vi "QMH-Check Loop Error.vi"(6 "Exit on Error? (F)":bool, 9 "Ignore Errors":i32[](array[numeric]), 10 "error to process":errorcluster, 11 "Message Queue":refnum<queue>) -> (2 "Error?":bool, 3 "dup Message Queue":refnum<queue>)   [LabVIEW 2019, in "Personalities Tool.lvlib"]
doc: "Check the 'error to process' to see if its code value matches any of the values in the 'Ignore Errors' array. If so, do nothing. If not, send an \"Error\" message containing the error data to the Message Handling Loop for further processing. If the \"Exit on Error?\" input is TRUE, send an \"Exit\" message to the Message Handling Loop instead."
uses:
  Personalities Tool.lvlib
  Message Cluster.ctl
  Enqueue Message (Single).vi
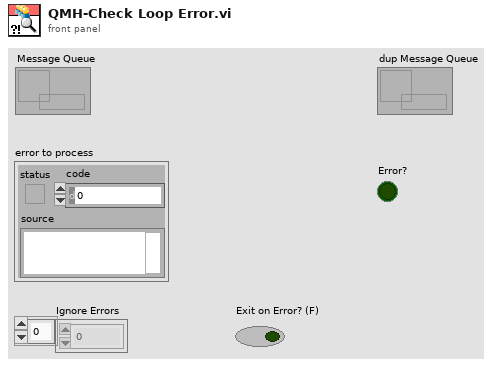
[diagram p1: front panel]
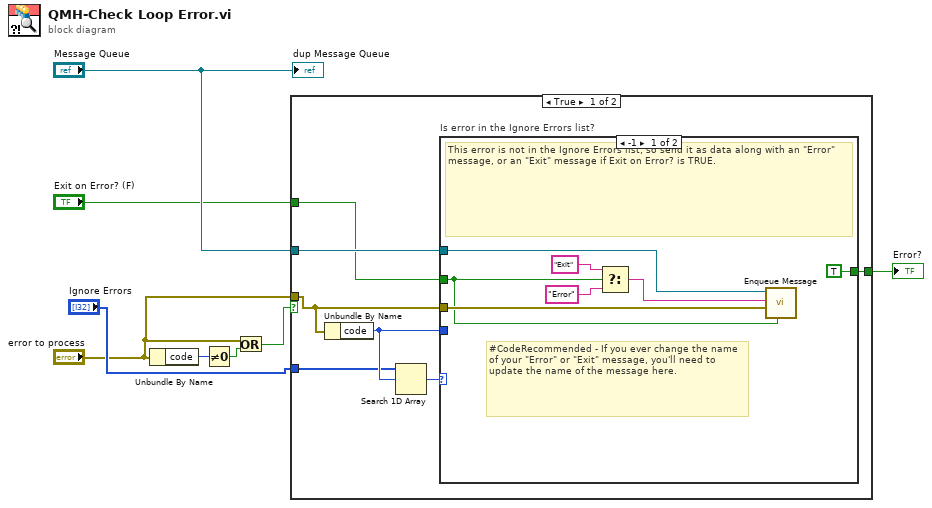
[diagram p0: block diagram]
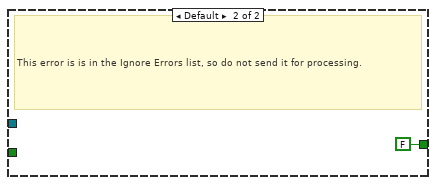
[diagram p2: hidden frame]
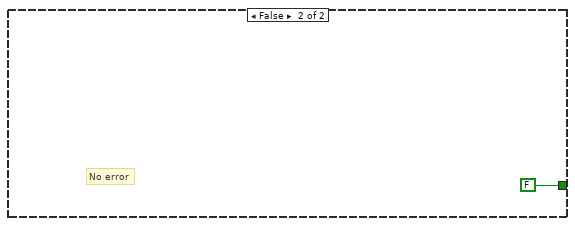
[diagram p3: hidden frame]
diagram:
  n1 = Unbundle By Name("error to process") -> ("code"=w2:i32)
  n2 = Not Equal To 0?(x=w2) -> (x != 0?=w1:bool)
  n3 = Or(x="error to process", y=w1) -> (x .or. y?=w4:bool)
  n4 = case shown="True" w4 {
    tunnel: "Message Queue" -> [w15 _]
    tunnel: "Ignore Errors" -> [w12 _]
    tunnel: [w11 FALSE] -> w6
    tunnel: "Exit on Error? (F)" -> [w10 _]
    tunnel: "error to process" -> [w9 _]
    frame True {
      n5 = Unbundle By Name(w9) -> ("code"=w13:i32)
      n6 = Search 1D Array(1D array=w12, element=w13) -> (index of element=w14:i32)  [unwired: 1 in]
      n7 = case "Is error in the Ignore Errors list?" shown="-1" w14 {
        tunnel: w9 -> [w20 _]
        tunnel: w15 -> [w22 _]
        tunnel: w13 -> [_ _]
        tunnel: [TRUE FALSE] -> w11
        tunnel: w10 -> [w19 _]
        frame -1 {
          # "#CodeRecommended - If you ever change the name of your \"Error\" or \"Exit\" message, you'll need to update the name of the message here."
          # "This error is not in the Ignore Errors list, so send it as data along with an \"Error\" message, or an \"Exit\" message if Exit on Error? is TRUE."
          n8 = Select(t="Exit" ("Message"), s=w19, f="Error" ("Message")) -> (s? t:f=w18:string)
          n9 = call-poly "Enqueue Message.vi"("Priority Message? (F)"=w19, "Message Data"=w20, "Message"=w18, "Message Queue"=w22) -> ()  [unwired: 6 in, 2 out]
        }
        frame Default {
          # "This error is is in the Ignore Errors list, so do not send it for processing."
        }
      }
    }
    frame False {
      # "No error"
    }
  }
  "Error?" <- w6
  "dup Message Queue" <- "Message Queue"
